vi "add_CameraControl.vi"(4 "Camera Control":cluster{"id":i32, "value":i32}, 5 "msg in":string) -> (2 "msg out":string)   [LabVIEW 2013]
uses:
  Primitives/subs/i32Scalar.vi
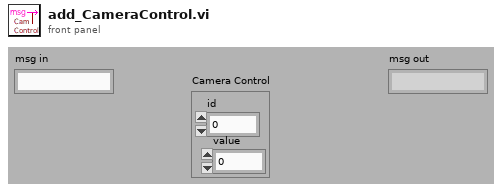
[diagram p1: front panel]
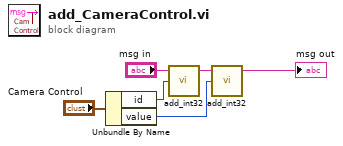
[diagram p0: block diagram]
diagram:
  n1 = Unbundle By Name("Camera Control") -> ("id"=w4:i32, "value"=w3:i32)
  n2 = call-poly "add_int32.vi"("Numeric"=w4, "msg in"="msg in") -> ("msg out"=w6:string)  [unwired: 3 in]
  n3 = call-poly "add_int32.vi"("Numeric"=w3, "msg in"=w6) -> ("msg out"=→"msg out":string)  [unwired: 3 in]
